vi "Append Error Details.vi"(0 "functionbase in":refnum<class "functionbase.lvclass">, 11 "error in (no error)":errorcluster) -> (4 "functionbase out":refnum<class "functionbase.lvclass">, 15 "error out":errorcluster)   [LabVIEW 2019, in "LSL.lvlib" / "functionbase.lvclass"]
uses:
  functionbase.lvclass
  common/function utils/Validate_message.ctl
  common/function utils/Validate_MessageStatus.ctl
  functionbase.lvclass/functionbase.ctl
  properties/Read Output Terminal.vi
  properties/Read Line#.vi
  properties/Write Output Terminal.vi
  output terminal/Base/Output Terminal.lvclass
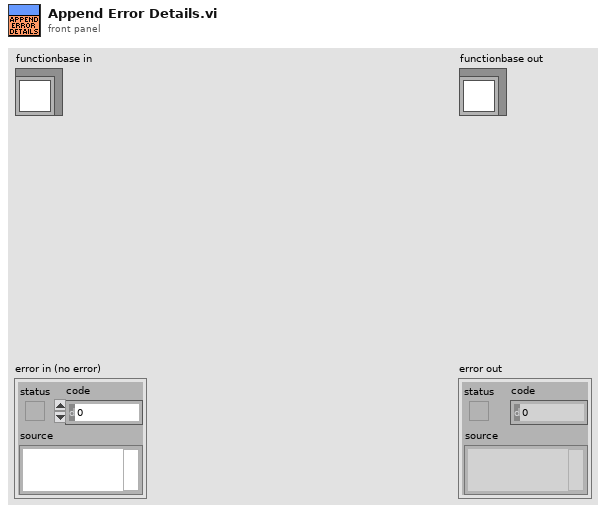
[diagram p1: front panel]
types:
  T1 = typedef "Validate_message.ctl" = cluster{"Line Number":i64, "Type":T2, "Message":string}
  T2 = typedef "Validate_MessageStatus.ctl" = enum16{"Message", "Warning", "Error"}
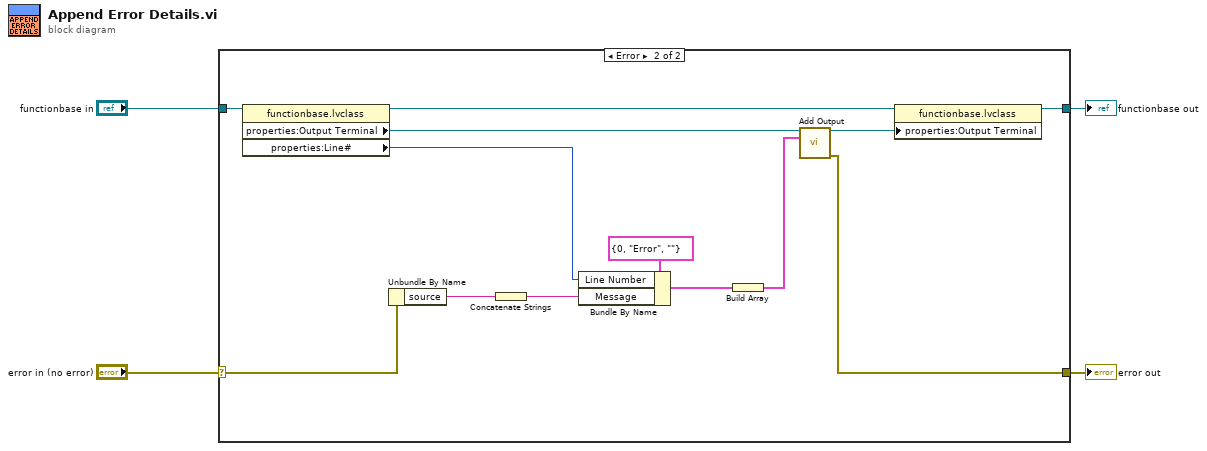
[diagram p0: block diagram]
diagram:
  n1 = case shown="Error" "error in (no error)" {
    selector: "error in (no error)" -> [w5 w19]
    tunnel: [w5 w16] -> w3
    tunnel: [w6 w14] -> w1
    tunnel: "functionbase in" -> [w6 w18]
    frame No Error {
    }
    frame Error {
      n2 = property class="functionbase.lvclass"(reference=w18) -> (reference out=w15:refnum<class "functionbase.lvclass">, "properties:Output Terminal"=w17:refnum<class "Output Terminal.lvclass">, "properties:Line#"=w11:i64)  [unwired: 1 in, 1 out]
      n3 = Unbundle By Name(w19) -> ("source"=w10:string)
      n4 = Concatenate Strings(w10) -> (w7:string)
      n5 = Bundle By Name(cluster=T1 {"Line Number"=0, "Type"=enum."Error", "Message"=""} ("Message"), "Line Number"=w11, "Message"=w7) -> (w9:T1)
      n6 = Build Array(w9) -> (w8:T1[])
      n7 = call-dynamic "Add Output.vi"("Output Terminal in"=w17, "Comiplation message"=w8) -> ("Output Terminal out"=w13:refnum<class "Output Terminal.lvclass">, "error out"=w16:errorcluster)  [unwired: 12 in]
      n8 = property class="functionbase.lvclass"(reference=w15, "properties:Output Terminal"=w13) -> (reference out=w14:refnum<class "functionbase.lvclass">)  [unwired: 1 in, 1 out]
    }
  }
  "error out" <- w3
  "functionbase out" <- w1
